vi "testLoopback.vi"(8 "error in (no error)":errorcluster, 11 "TestCase in":refnum<class "SLSC 12201 System Tests.lvclass">) -> (0 "error out":errorcluster, 3 "TestCase out":refnum<class "SLSC 12201 System Tests.lvclass">)   [LabVIEW 2020, in "SLSC 12201 System Tests.lvclass"]
uses:
  SLSC 12201 System Tests.lvclass
  C:/Program Files (x86)/National Instruments/LabVIEW 2020/vi.lib/NI/VeriStand Custom Device Testing Tools/VeriStandTestCase/VeriStandTestCase.lvclass
  C:/Program Files (x86)/National Instruments/LabVIEW 2020/vi.lib/addons/_JKI Toolkits/VI Tester/TestCase.llb/TestCase.lvclass
  Loopback/Loopback.lvclass
  <vilib>/addons/_JKI Toolkits/VI Tester/TestCase.llb/TestCase.lvclass
  <vilib>/NI/VeriStand Custom Device Testing Tools/VeriStandTestCase/VeriStandTestCase.lvclass
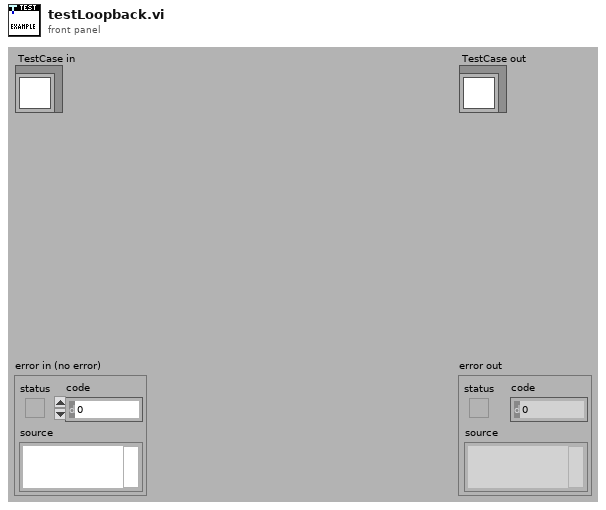
[diagram p1: front panel]
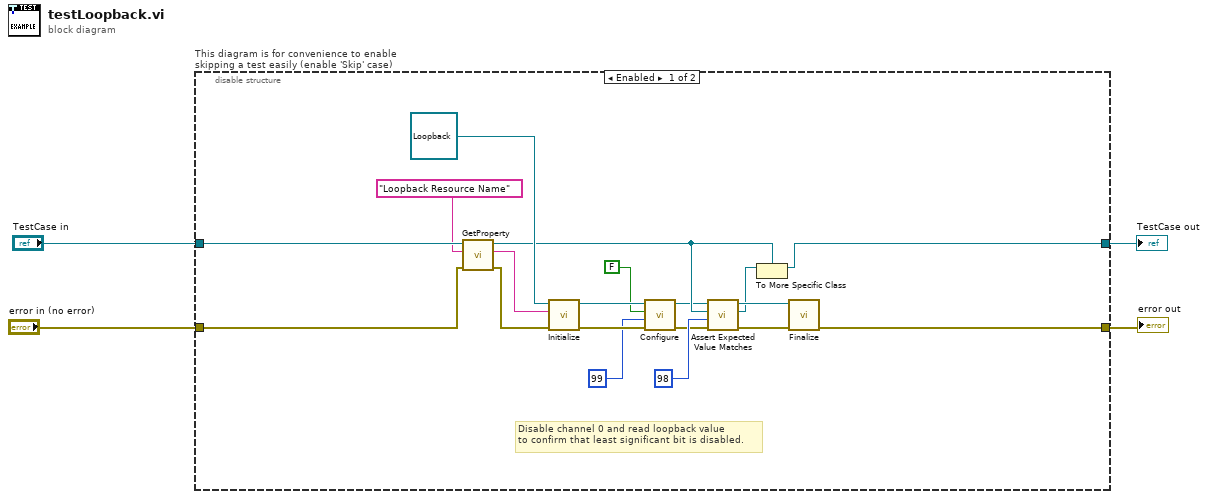
[diagram p0: block diagram]
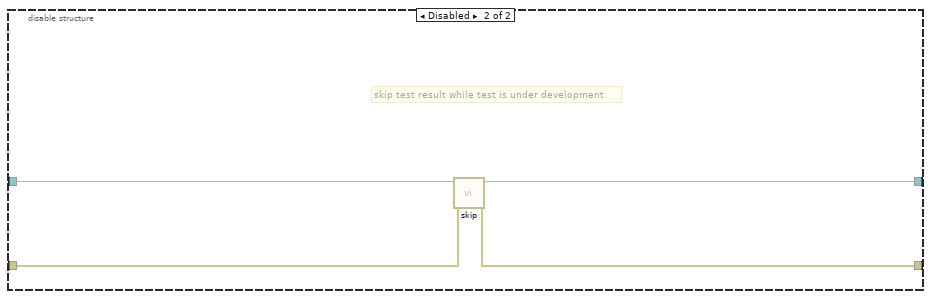
[diagram p2: hidden frame]
diagram:
  n1 = disable-structure "This diagram is for convenience to enable skipping a test easily (enable 'Skip' case)" shown="Enabled" {
    disable-tunnel: "TestCase in" -> [w23 w27]
    disable-tunnel: [w9 w25] -> w1
    disable-tunnel: [w20 w26] -> w3
    disable-tunnel: "error in (no error)" -> [w6 w24]
    frame Enabled {
      # "Disable channel 0 and read loopback value\nto confirm that least significant bit is disabled."
      n2 = call <vilib>:"GetProperty.vi"("error in (no error)"=w6, "key"="Loopback Resource Name", "VeriStandTestCase in"=w23) -> ("error out"=w5:errorcluster, "value"=w18:string, "VeriStandTestCase out"=w16:refnum<class "SLSC 12201 System Tests.lvclass">)  [unwired: 6 in]
      n3 = call-dynamic "Initialize.vi"("error in (no error)"=w5, "Resource Name in"=w18, "Loopback in"=refnum<class "Loopback.lvclass"> refnum ("Loopback.lvclass")) -> ("error out"=w21:errorcluster, "Loopback out"=w17:refnum<class "Loopback.lvclass">)  [unwired: 7 in]
      n4 = call-dynamic "Configure.vi"("error in (no error)"=w21, "Value in"=u8 99, "Use Counter?"=FALSE, "Loopback in"=w17) -> ("error out"=w8:errorcluster, "Loopback out"=w15:refnum<class "Loopback.lvclass">)  [unwired: 6 in]
      n5 = call-dynamic "Assert Expected Value Matches.vi"("error in (no error)"=w8, "Expected Value"=u8 98, "TestCase in"=w16, "Loopback in"=w15) -> ("error out"=w7:errorcluster, "TestCase out"=w10:refnum<class "TestCase.lvclass">, "Loopback out"=w12:refnum<class "Loopback.lvclass">)  [unwired: 5 in]
      n6 = To More Specific Class(target class=w16, reference=w10) -> (specific class reference=w9:refnum<class "SLSC 12201 System Tests.lvclass">)  [unwired: 1 in, 1 out]
      n7 = call-dynamic "Finalize.vi"("error in (no error)"=w7, "Loopback in"=w12) -> ("error out"=w20:errorcluster)  [unwired: 8 in, 1 out]
    }
    frame Disabled {
      # "skip test result while test is under development"
      n8 = call <vilib>:"skip.vi"("error in (no error)"=w24, "TestCase in"=w27) -> ("error out"=w26:errorcluster, "TestCase out"=w25:refnum<class "SLSC 12201 System Tests.lvclass">)  [unwired: 8 in]
    }
  }
  "error out" <- w3
  "TestCase out" <- w1
